vi "CAN_Close.vi"(8 "error in (no error)":errorcluster caption="错误输入（无错误）", 11 "General_Input":T1={"DevType"=1, "DevIndex"=0, "CANIndex"=0} {"CANIndex" items=["0", "1"]; "DevType" items=["PCI5121"=1, "PCI9810"=2, "USBCAN1"=3, "USBCAN2"=4, "PCI9820"=5, "CAN232"=6, "PCI5110"=7, "CANLite(mini)"=8, "ISA9620"=9, "ISA5420"=10, "PC104CAN"=11, "CANETE"=12, "DNP9810"=13, "PCI9840B"=14, "PC104C2"=15, "PCI9820I"=16]}) -> (0 "error out":errorcluster caption="错误输出", 2 "CloseOrNot":u32)   [LabVIEW 2012]
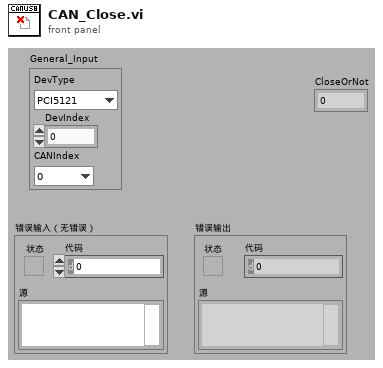
[diagram p1: front panel]
types:
  T1 = cluster{"DevType":u16, "DevIndex":u32, "CANIndex":u16}
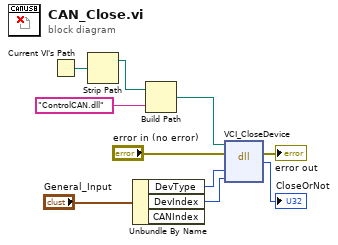
[diagram p0: block diagram]
diagram:
  n1 = Current VI's Path() -> (path=w6:path)
  n2 = Strip Path(path=w6) -> (stripped path=w7:path)  [unwired: 1 out]
  n3 = Unbundle By Name("General_Input") -> ("DevType"=w3:u16, "DevIndex"=w2:u32)  [unwired: 1 out]
  n4 = Build Path(base path=w7, name or relative path="ControlCAN.dll" ("名称或相对路径")) -> (appended path=w4:path)
  n5 = dll-call lib="?" fn="VCI_CloseDevice"(path in=w4, error in="error in (no error)", "DevType"=w3, "DevIndex"=w2) -> (error out=→"error out":errorcluster, "CloseOrNot"=→"CloseOrNot":u32)  [unwired: 3 in, 1 out]
